vi "LowWrite.vi"(5 "LogSuspend":bool, 8 "error in":errorcluster, 9 "Messages":T3[](array[typedef]), 10 "Number to Write":i32, 11 "UdsHandleIn":T1={"LogPath"=path "", "LogEnabled"=FALSE, "isOpen"=FALSE, "LogContent"="", "Adapter"="CAN0", "MCanHandle"={"MCanAdapter"=refnum}, "TransmittId"=0, "ReceiveId"=0}) -> (0 "error out":errorcluster, 3 "UdsHandleOut":T1={"LogPath"=path "", "LogEnabled"=FALSE, "isOpen"=FALSE, "LogContent"="", "Adapter"="CAN0", "MCanHandle"={"MCanAdapter"=refnum}, "TransmittId"=0, "ReceiveId"=0})   [LabVIEW 2011, in "Konvolucio MUDS150628.lvlib"]
uses:
  <instrlib>/Konvolucio MUDS150628/Konvolucio MUDS150628.lvlib
  <instrlib>/Konvolucio MCAN120803/Types/MessageType.ctl
  <instrlib>/Konvolucio MUDS150628/Types/UdsHandleType.ctl
  <instrlib>/Konvolucio MCAN120803/Types/MCanHandleType.ctl
  C:/Program Files/National Instruments/LabVIEW 2011/instr.lib/Konvolucio MCAN120803/Private/Konvolucio.MCAN120803.dll
  Konvolucio MCAN120803/Private/Konvolucio.MCAN120803.dll
  <instrlib>/Konvolucio MUDS150628/Private/UdsLogCanTxMessage.vi
  <instrlib>/Konvolucio MCAN120803/Konvolucio MCAN120803.lvlib
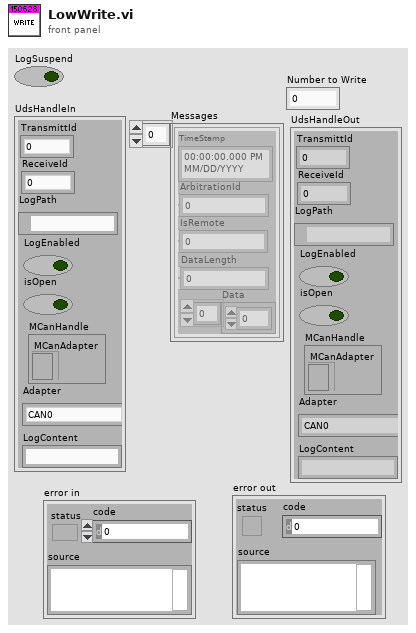
[diagram p1: front panel]
types:
  T1 = typedef "Konvolucio MUDS150628.lvlib/UdsHandleType.ctl" = cluster{"LogPath":path, "LogEnabled":bool, "isOpen":bool, "LogContent":string, "Adapter":string, "MCanHandle":T2, "TransmittId":u32, "ReceiveId":u32}
  T2 = typedef "Konvolucio MCAN120803.lvlib/MCanHandleType.ctl" = cluster{"MCanAdapter":refnum<k24>}
  T3 = typedef "Konvolucio MCAN120803.lvlib/MessageType.ctl" = cluster{"TimeStamp":timestamp, "ArbitrationId":u32, "IsRemote":u8, "DataLength":u8, "Data":u8[]}
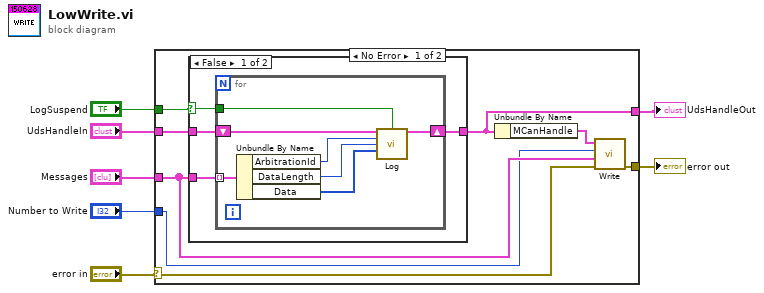
[diagram p0: block diagram]
diagram:
  n1 = case shown="No Error" "error in" {
    selector: "error in" -> [w9 w28]
    tunnel: "LogSuspend" -> [w15 _]
    tunnel: "UdsHandleIn" -> [w14 w29]
    tunnel: "Messages" -> [w13 _]
    tunnel: "Number to Write" -> [w12 _]
    tunnel: [w10 w28] -> w3
    tunnel: [w8 w29] -> w2
    frame No Error {
      n2 = case shown="False" w15 {
        selector: w15 -> [w16 _]
        tunnel: w13 -> [w19 _]
        tunnel: w14 -> [w18 w27]
        tunnel: [w17 w27] -> w8
        frame False {
          n3 = for {
            shift-right: [w24] -> w17
            shift-left: w18 -> [w25]
            tunnel: w19 -> [w26] mode=indexing
            tunnel: w16 -> [w23]
            n4 = Unbundle By Name(w26) -> ("ArbitrationId"=w22:u32, "DataLength"=w21:u8, "Data"=w20:u8[])
            n5 = call-poly <instrlib>:"Log.vi"("UdsHandleIn"=w25, "LogSuspend"=w23, "Id"=w22, "DataLength"=w21, "Data"=w20) -> ("UdsHandleOut"=w24:T1)  [unwired: 9 in, 1 out]
          }
        }
        frame True {
        }
      }
      n6 = Unbundle By Name(w8) -> ("MCanHandle"=w11:T2)
      n7 = call <instrlib>:"Write.vi"("error in"=w9, "Messages"=w13, "Number to Write"=w12, "MCanHandleIn"=w11) -> ("error out"=w10:errorcluster)  [unwired: 4 in, 1 out]
    }
    frame Error {
    }
  }
  "error out" <- w3
  "UdsHandleOut" <- w2
